vi "Display.vi"() -> ()   [LabVIEW 2020]
panel:
  out "High temperature":bool
  out "Trend":dbl
  out "TimeDisplay":string
  out "TempChart":dbl(graph)
  in  "Stop":bool
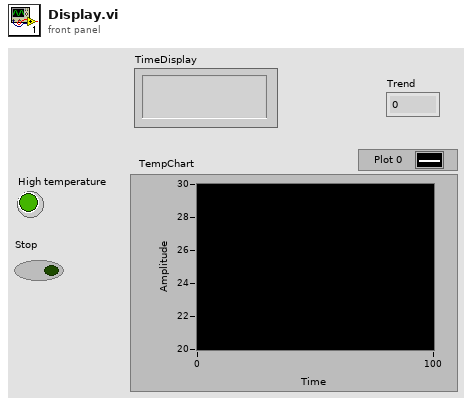
[diagram p1: front panel]
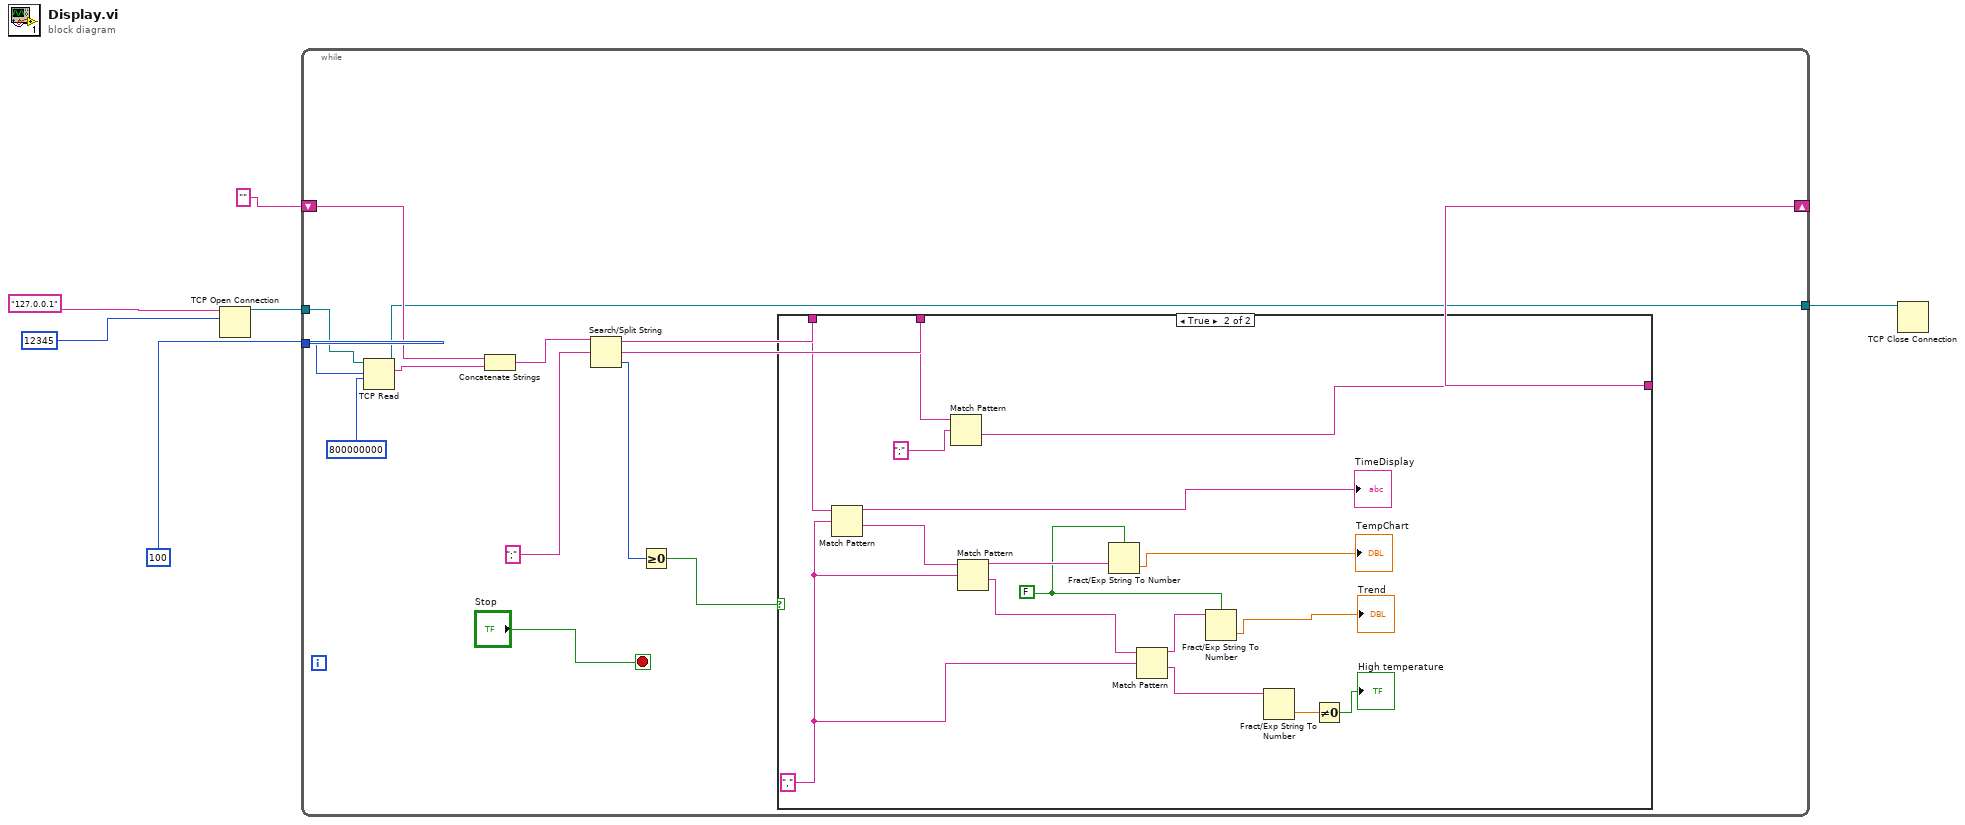
[diagram p0: block diagram]
diagram:
  n1 = TCP Open Connection(address="127.0.0.1", remote port or service name=12345) -> (connection ID=w5:refnum<k5>)  [unwired: 3 in, 1 out]
  n2 = while {
    tunnel: w5 -> [w10]
    tunnel: 100 -> [w11]
    tunnel: [w8] -> w3
    shift-right: [w14] -> _
    shift-left: "" -> [w19]
    stop <- "Stop" stop-if-true
    n3 = TCP Read(connection ID=w10, bytes to read=w11, 9:800000000) -> (connection ID out=w8:refnum<k5>, data out=w9:string)  [unwired: 2 in, 1 out]
    n4 = Concatenate Strings(w19, w9) -> (w17:string)
    n5 = Search/Split String(string=w17, search string/char (-)=";") -> (substring before match=w13:string, match + rest of string=w12:string, offset of match=w16:i32)  [unwired: 1 in]
    n6 = Greater Or Equal To 0?(x=w16) -> (x >= 0?=w15:bool)
    n7 = case shown="True" w15 {
      tunnel: [w21 w33] -> w14
      tunnel: w13 -> [w21 w36]
      tunnel: w12 -> [_ w34]
      frame False {
      }
      frame True {
        w28 = FALSE
        w27 = ","
        n8 = Match Pattern(string=w36, regular expression=w27) -> (before substring=→"TimeDisplay":string, after substring=w32:string)  [unwired: 1 in, 2 out]
        n9 = Match Pattern(string=w34, regular expression=";") -> (after substring=w33:string)  [unwired: 1 in, 3 out]
        n10 = Match Pattern(string=w32, regular expression=w27) -> (before substring=w31:string, after substring=w26:string)  [unwired: 1 in, 2 out]
        n11 = Fract/Exp String To Number(use system decimal point (T)=w28, string=w31) -> (number=→"TempChart":dbl)  [unwired: 2 in, 1 out]
        n12 = Match Pattern(string=w26, regular expression=w27) -> (before substring=w25:string, after substring=w24:string)  [unwired: 1 in, 2 out]
        n13 = Fract/Exp String To Number(use system decimal point (T)=w28, string=w25) -> (number=→"Trend":dbl)  [unwired: 2 in, 1 out]
        n14 = Fract/Exp String To Number(string=w24) -> (number=w22:dbl)  [unwired: 3 in, 1 out]
        n15 = Not Equal To 0?(x=w22) -> (x != 0?=→"High temperature":bool)
      }
    }
  }
  n16 = TCP Close Connection(connection ID=w3) -> ()  [unwired: 2 in, 2 out]
